vi "VI1.vi"() -> ()   [LabVIEW 2020]
uses:
  <vilib>/Utility/NIReport.llb/Report Type.ctl
  <vilib>/DAQmx/write.llb/DAQmx Write (Analog Wfm 1Chan NSamp).vi
  <vilib>/DAQmx/read.llb/DAQmx Read (Analog 1D Wfm NChan NSamp).vi
  <vilib>/DAQmx/miscellaneous.llb/DAQmx Fill In Error Info.vi
  <vilib>/measure/madcrms.llb/Basic Averaged DC-RMS for 1 Chan.vi
  <vilib>/Utility/NIReport.llb/Append Report Text (str wrap).vi
  <vilib>/measure/mascope.llb/Amplitude and Levels 1 chan.vi
  <vilib>/Utility/NIReport.llb/NI_report.lvclass
  <vilib>/measure/NI_MABase.lvlib
  <vilib>/measure/NI_MAPro.lvlib
  <vilib>/Utility/NIReport.llb/NI_ReportGenerationCore.lvlib
panel:
  in  "Tab Control 2":T1(tab)
  out "input signal":waveform(dbl)(graph)
  out "output signal":waveform(dbl)(graph)
  out "DC input":dbl format="%0.2p"
  out "RMS input":dbl format="%0.2p"
  out "DC output":dbl format="%0.2p"
  out "RMS output":dbl format="%0.2p"
  in  "amplitude 2":dbl=1.0 format="%0.2p"
  in  "rate 2":dbl=1000.0
  in  "number of samples 2":dbl=100.0
  in  "frequency":dbl=10.0 format="%0.2p"
  in  "offset":dbl format="%0.2p"
  out "iter":i32
  out "N\n 2":i32=100
  in  "(1) student ID 2":string
  in  "(1) student name  2":string
  in  "(1) student name":string
  in  "(1) student ID":string
  out "Date and time 8":string
  in  "(1) additional comment":string
  out "common gain":cluster{dbl[], dbl[]}(graph)
  out "ch 1 signal":waveform(dbl)(graph)
  out "ch 2 signal":waveform(dbl)(graph)
  in  "amplitude 3":dbl=1.0 format="%0.2p"
  in  "offset 2":dbl format="%0.2p"
  in  "Rprobe":dbl format="%0.2p"
  in  "To   [Hz]":i32
  in  "From [Hz]":dbl
  in  "jump":dbl=1.0 format="%#_13g"
  out "current freq":dbl
  in  "rate 3":dbl=1000.0
  in  "number of samples 3":dbl=100.0
  out "current jump":dbl=1.0
  out "N 4":dbl
  out "i 4":i32
  out "ch 1 input":waveform(dbl)(graph)
  out "ch 0 output":waveform(dbl)(graph)
  in  "jump [volt]":dbl=1.0 format="%#_13g"
  in  "From [volt]":dbl
  out "current amp":dbl
  in  "To   [volt]":i32
  in  "rate 7":dbl=1000.0
  in  "number of samples 7":dbl=100.0
  out "current jump 2":dbl=1.0
  in  "offset 3":dbl format="%0.2p"
  in  "frequency 2":dbl=10.0 format="%0.2p"
  out "N 7":dbl
  out "i 7":i32
  out "Vpp ch0":dbl format="%.2p"
  out "Vpp ch1":dbl format="%.2p"
  in  "stop":bool
  out "Date and time 7":string
  in  "(7) student ID 1":string
  in  "(7) student name 1":string
  in  "(7) student name 2":string
  in  "(7) student ID 2":string
  in  "(7) additional comment":string
  out "start volt 2":dbl
  # "offset measurment"
  # "function generator"
  # "Report generation"
  # "measurment details"
  # "frequency sweep"
  # "function generator"
  # "Dynamic range measurment"
  # "voltage sweep"
  # "function generator"
  # "Report generation"
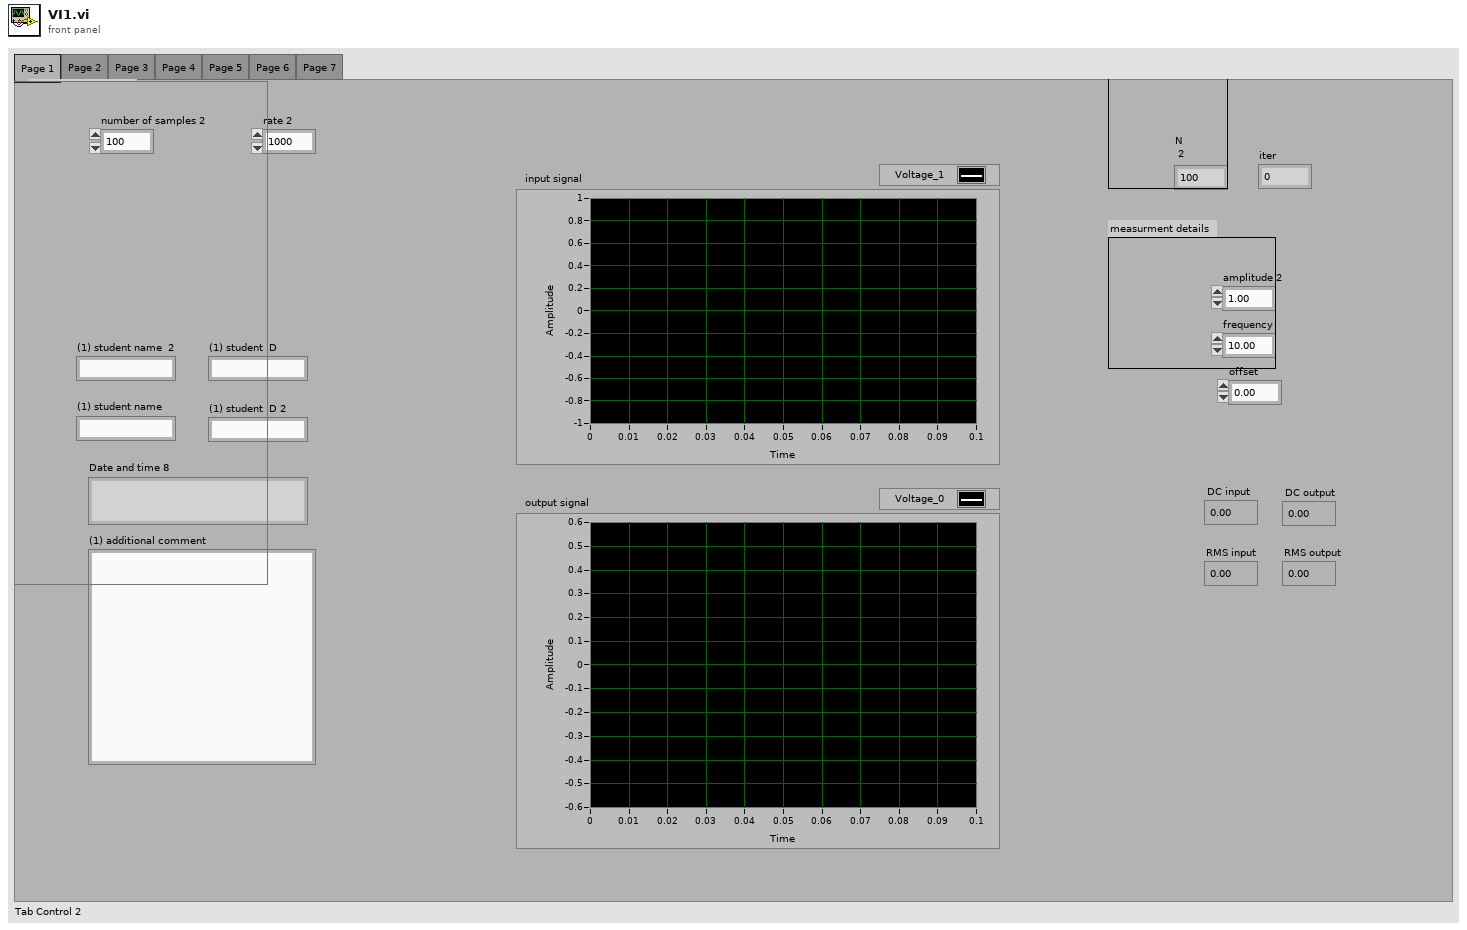
[diagram p1: front panel]
types:
  T1 = enum32{"Page 1", "Page 2", "Page 3", "Page 4", "Page 5", "Page 6", "Page 7"}
  T2 = typedef "NI_ReportGenerationCore.lvlib/Report Type.ctl" = enum16{"HTML", "Word", "Excel"}
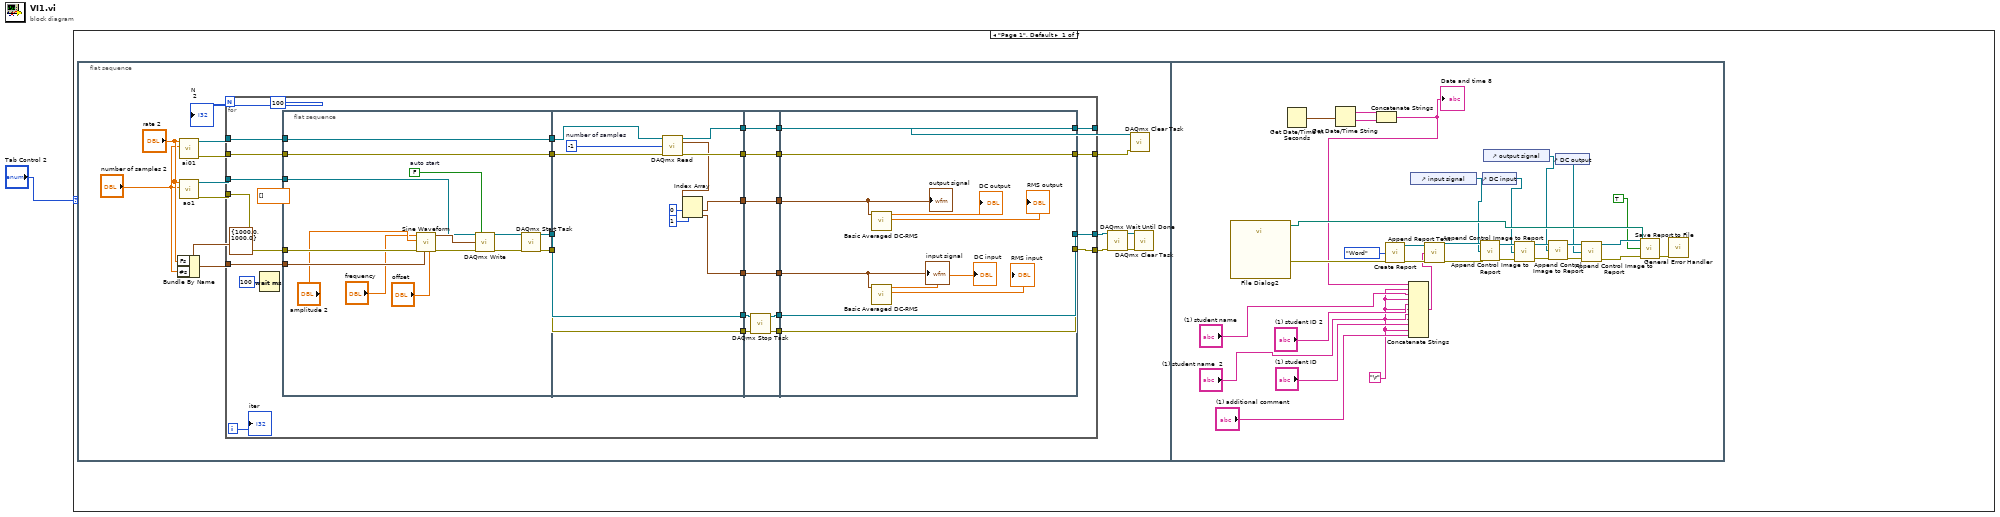
[diagram p0: block diagram]
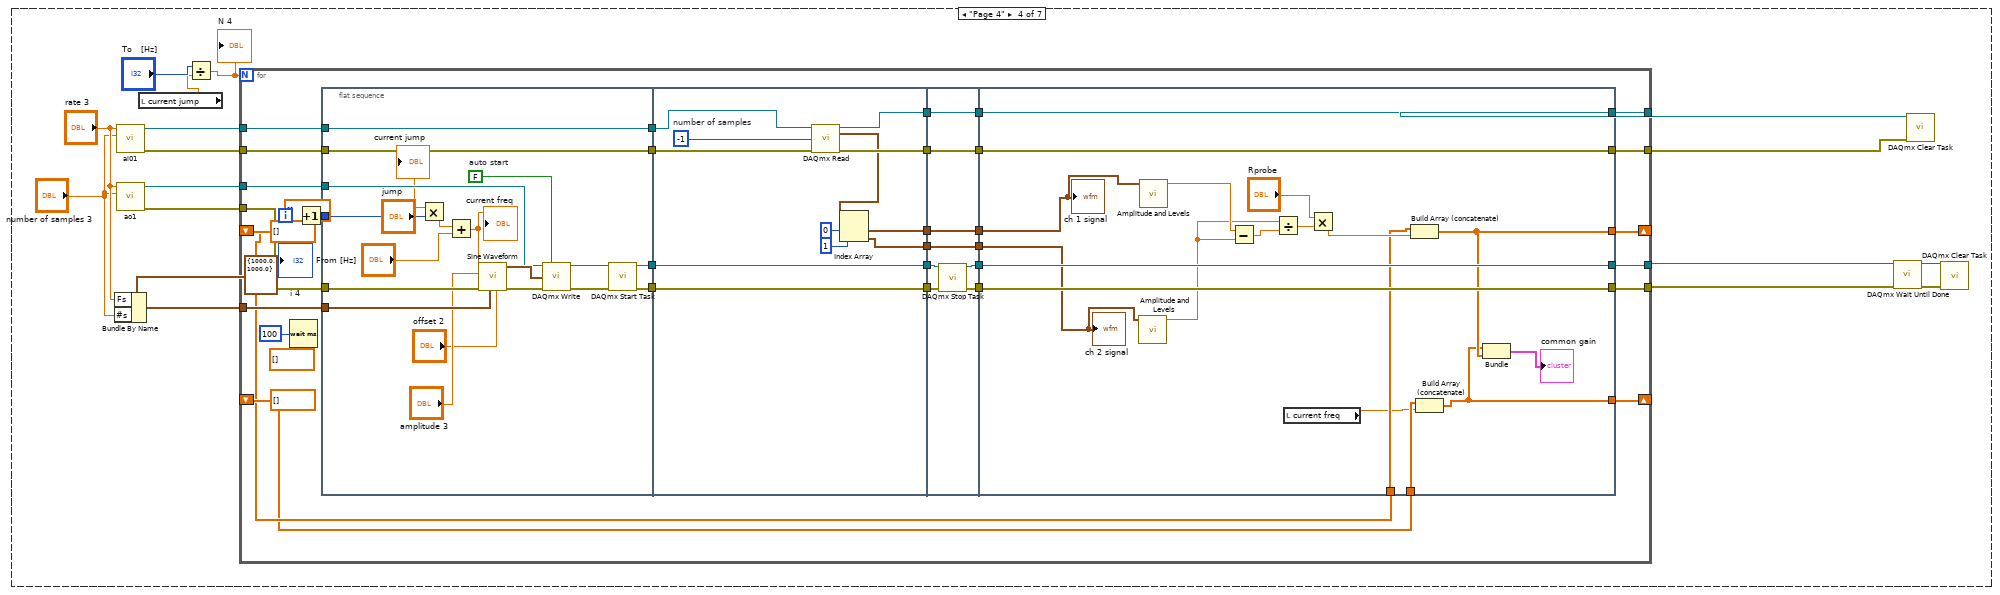
[diagram p4: hidden frame]
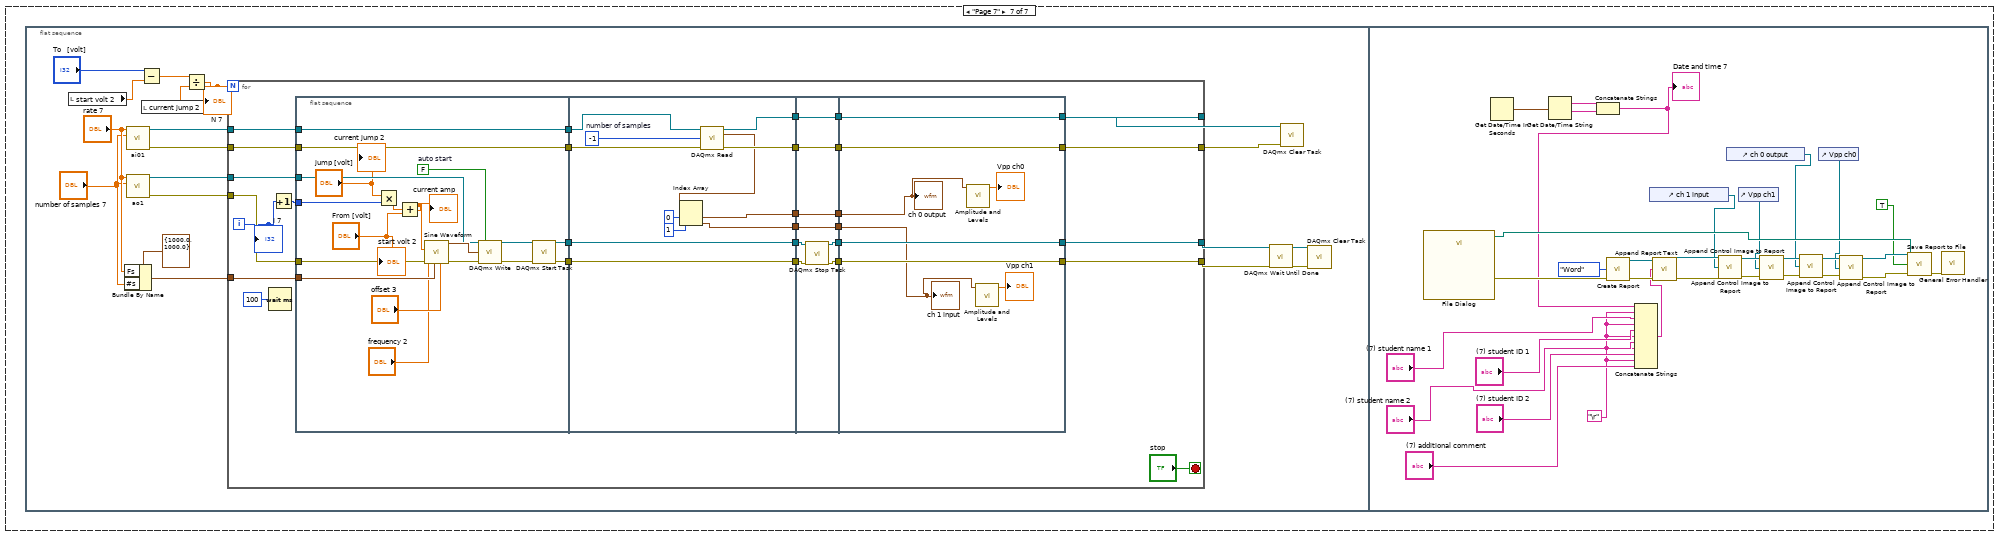
[diagram p7: hidden frame]
diagram:
  n1 = case shown="\"Page 1\", Default" "Tab Control 2" {
    frame "Page 1", Default {
      n2 = flat-sequence {
        frame #0 {
          (unwired) dbl[] []
          w10 = 100
          n3 = Bundle By Name(cluster=cluster{"Fs":dbl, "#s":dbl} {"Fs"=1000.0, "#s"=1000.0} ("sampling info"), "Fs"="rate 2", "#s"="number of samples 2") -> (w11:cluster{"Fs":dbl, "#s":dbl})
          n4 = call "ai01.vi"("number of samples"="number of samples 2", "rate"="rate 2") -> ("error out"=w6:errorcluster, "task out"=w7:refnum<k21>)  [unwired: 8 in]
          n5 = call "ao1.vi"("number of samples"="number of samples 2", "rate"="rate 2") -> ("error out"=w14:errorcluster, "task out"=w13:refnum<k21>)  [unwired: 8 in]
          n6 = for {
            N: w10 -> [_]
            tunnel: w14 -> [w43]
            tunnel: w13 -> [w42]
            tunnel: w11 -> [w41]
            tunnel: [w40] -> w9
            tunnel: [w39] -> w8
            tunnel: w7 -> [w38]
            tunnel: w6 -> [w36]
            tunnel: [w33] -> w3
            tunnel: [w31] -> w2
            i -> [w17]
            n7 = Wait (ms)(milliseconds to wait=u32 100) -> ()  [unwired: 1 out]
            n8 = flat-sequence {
              tunnel: w43 -> [w55]
              tunnel: w42 -> [w54]
              tunnel: w41 -> [w53]
              tunnel: w38 -> [w49]
              tunnel: [w49] -> w37
              tunnel: w36 -> [w48]
              tunnel: [w48] -> w35
              tunnel: [w47] -> w29
              tunnel: [w46] -> w27
              tunnel: w37 -> [w69]
              tunnel: w35 -> [w68]
              tunnel: [w67] -> w34
              tunnel: [w66] -> w32
              tunnel: [w65] -> w30
              tunnel: w29 -> [w65]
              tunnel: [w64] -> w28
              tunnel: w27 -> [w64]
              tunnel: [w60] -> w20
              tunnel: [w59] -> w18
              tunnel: w34 -> [w76]
              tunnel: w32 -> [w75]
              tunnel: w30 -> [w74]
              tunnel: w28 -> [w73]
              tunnel: [w78] -> w25
              tunnel: [w77] -> w24
              tunnel: [w76] -> w23
              tunnel: [w75] -> w22
              tunnel: [w72] -> w21
              tunnel: w20 -> [w72]
              tunnel: [w71] -> w19
              tunnel: w18 -> [w71]
              tunnel: [w85] -> w31
              tunnel: [w86] -> w33
              tunnel: [w87] -> w39
              tunnel: [w88] -> w40
              tunnel: w25 -> [w88]
              tunnel: w24 -> [w87]
              tunnel: w23 -> [w86]
              tunnel: w22 -> [w85]
              tunnel: w21 -> [w84]
              tunnel: w19 -> [w83]
              frame #0 {
                w58 = FALSE  # auto start
                n9 = call <vilib>:"Sine Waveform.vi"("offset"="offset", "sampling info"=w53, "error in (no error)"=w55, "amplitude"="amplitude 2", "frequency"="frequency") -> ("error out"=w57:errorcluster, "signal out"=w56:waveform(dbl))  [unwired: 5 in]
                n10 = call-poly <vilib>:"DAQmx Write.vi"("task/channels in"=w54, "auto start"=w58, "data"=w56, "error in"=w57) -> ("task out"=w51:refnum<k21>, "error out"=w50:errorcluster)  [unwired: 9 in, 1 out]
                n11 = call <vilib>:"DAQmx Start Task.vi"("task/channels in"=w51, "error in"=w50) -> ("task out"=w47:refnum<k21>, "error out"=w46:errorcluster)  [unwired: 12 in]
              }
              frame #1 {
                w70 = -1  # number of samples
                n12 = call-poly <vilib>:"DAQmx Read.vi"("task/channels in"=w69, "number of samples per channel"=w70, "error in"=w68) -> ("task out"=w67:refnum<k21>, "data"=w63:waveform(dbl)[], "error out"=w66:errorcluster)  [unwired: 10 in]
                n13 = Index Array(array=w63, index #1=0 ("index"), index #2=1 ("index")) -> (element #1=w60:waveform(dbl), element #2=w59:waveform(dbl))
              }
              frame #2 {
                n14 = call <vilib>:"DAQmx Stop Task.vi"("task/channels in"=w74, "error in"=w73) -> ("task out"=w78:refnum<k21>, "error out"=w77:errorcluster)  [unwired: 12 in]
              }
              frame #3 {
                n15 = call-poly <vilib>:"Basic Averaged DC-RMS.vi"("signal in"=w84) -> ("RMS value"=→"RMS output":dbl, "DC value"=→"DC output":dbl)  [unwired: 7 in, 2 out]
                n16 = call-poly <vilib>:"Basic Averaged DC-RMS.vi"("signal in"=w83) -> ("RMS value"=→"RMS input":dbl, "DC value"=→"DC input":dbl)  [unwired: 7 in, 2 out]
                "output signal" <- w84
                "input signal" <- w83
              }
            }
            "iter" <- w17
          }
          n17 = call <vilib>:"DAQmx Wait Until Done.vi"("task/channels in"=w9, "error in"=w8) -> ("task out"=w15:refnum<k21>, "error out"=w16:errorcluster)  [unwired: 12 in]
          n18 = call <vilib>:"DAQmx Clear Task.vi"("task in"=w3, "error in"=w2) -> ()  [unwired: 13 in, 1 out]
          n19 = call <vilib>:"DAQmx Clear Task.vi"("task in"=w15, "error in"=w16) -> ()  [unwired: 13 in, 1 out]
          "N\n 2" <- w10
        }
        frame #1 {
          w105 = "\r"
          n20 = call "File Dialog2"() -> ("selected path"=w108:path, "error out"=w107:errorcluster)  [unwired: 12 in, 2 out]
          n21 = Get Date/Time In Seconds() -> (seconds since 1Jan1904=w120:timestamp)
          n22 = Get Date/Time String(seconds (now)=w120) -> (date string=w118:string, time string=w119:string)  [unwired: 2 in]
          n23 = Concatenate Strings(w118, w119) -> (w103:string)
          "Date and time 8" <- w103
          n24 = call <vilib>:"Create Report.vi"("report type"=Report_Type."Word", "error in (no error)"=w107) -> ("report out"=w109:refnum<class "NI_report.lvclass">, "error out"=w111:errorcluster)  [unwired: 12 in]
          n25 = Concatenate Strings(w103, w105, "(1) student name", w105, "(1) student ID 2", w105, "(1) student name  2", w105, "(1) student ID", w105, "(1) additional comment") -> (w101:string)
          n26 = control-ref of="input signal"() -> (w92:refnum<vi>)
          n27 = call-poly <vilib>:"Append Report Text.vi"("report in"=w109, "text"=w101, "error in (no error)"=w111) -> ("report out"=w94:refnum<class "NI_report.lvclass">, "error out"=w93:errorcluster)  [unwired: 9 in, 2 out]
          n28 = call-dynamic "Append Control Image to Report.vi"("report in"=w94, "ctrl reference"=w92, "error in (no error)"=w93) -> ("report out"=w96:refnum<class "NI_report.lvclass">, "error out"=w95:errorcluster)  [unwired: 9 in, 2 out]
          n29 = control-ref of="DC input"() -> (w91:refnum<vi>)
          n30 = control-ref of="output signal"() -> (w90:refnum<vi>)
          n31 = call-dynamic "Append Control Image to Report.vi"("report in"=w96, "ctrl reference"=w91, "error in (no error)"=w95) -> ("report out"=w97:refnum<class "NI_report.lvclass">, "error out"=w98:errorcluster)  [unwired: 9 in, 2 out]
          n32 = call-dynamic "Append Control Image to Report.vi"("report in"=w97, "ctrl reference"=w90, "error in (no error)"=w98) -> ("report out"=w100:refnum<class "NI_report.lvclass">, "error out"=w99:errorcluster)  [unwired: 9 in, 2 out]
          n33 = control-ref of="DC output"() -> (w89:refnum<vi>)
          n34 = call-dynamic "Append Control Image to Report.vi"("report in"=w100, "ctrl reference"=w89, "error in (no error)"=w99) -> ("report out"=w110:refnum<class "NI_report.lvclass">, "error out"=w112:errorcluster)  [unwired: 9 in, 2 out]
          n35 = call-dynamic "Save Report to File.vi"("report in"=w110, "report file path"=w108, "prompt to replace? (F)"=TRUE, "error in (no error)"=w112) -> ("error out"=w102:errorcluster)  [unwired: 10 in, 1 out]
          n36 = call <vilib>:"General Error Handler.vi"("error in (no error)"=w102) -> ()  [unwired: 10 in, 5 out]
        }
      }
    }
    frame "Page 2" {
    }
    frame "Page 3" {
    }
    frame "Page 4" {
      (unwired) dbl[] []
      (unwired) dbl[] []
      n37 = Bundle By Name(cluster=cluster{"Fs":dbl, "#s":dbl} {"Fs"=1000.0, "#s"=1000.0} ("sampling info"), "Fs"="rate 3", "#s"="number of samples 3") -> (w136:cluster{"Fs":dbl, "#s":dbl})
      n38 = call "ai01.vi"("number of samples"="number of samples 3", "rate"="rate 3") -> ("error out"=w134:errorcluster, "task out"=w135:refnum<k21>)  [unwired: 8 in]
      n39 = call "ao1.vi"("number of samples"="number of samples 3", "rate"="rate 3") -> ("error out"=w139:errorcluster, "task out"=w138:refnum<k21>)  [unwired: 8 in]
      n40 = local read "current jump"() -> (w125:dbl)
      n41 = Divide(x="To   [Hz]", y=w125) -> (x/y=w127:dbl)
      "N 4" <- w127
      n42 = for {
        N: w127 -> [_]
        tunnel: w139 -> [w171]
        tunnel: w138 -> [w170]
        tunnel: w136 -> [w167]
        tunnel: [w166] -> w122
        tunnel: [w165] -> w121
        tunnel: w135 -> [w164]
        tunnel: w134 -> [w162]
        tunnel: [w159] -> w131
        tunnel: [w157] -> w130
        shift-right: [w143] -> _
        shift-left: dbl[] [] -> [w142]
        shift-right: [w141] -> _
        shift-left: dbl[] [] -> [w140]
        i -> [w169]
        n43 = Wait (ms)(milliseconds to wait=u32 100) -> ()  [unwired: 1 out]
        n44 = Increment(x=w169) -> (x+1=w168:i32)
        n45 = flat-sequence {
          tunnel: w171 -> [w187]
          tunnel: w170 -> [w186]
          tunnel: w168 -> [w175]
          tunnel: w167 -> [w184]
          tunnel: w164 -> [w181]
          tunnel: [w181] -> w163
          tunnel: w162 -> [w180]
          tunnel: [w180] -> w161
          tunnel: [w179] -> w155
          tunnel: [w178] -> w153
          tunnel: w163 -> [w201]
          tunnel: w161 -> [w200]
          tunnel: [w199] -> w160
          tunnel: [w198] -> w158
          tunnel: [w197] -> w156
          tunnel: w155 -> [w197]
          tunnel: [w196] -> w154
          tunnel: w153 -> [w196]
          tunnel: [w192] -> w146
          tunnel: [w191] -> w145
          tunnel: w160 -> [w208]
          tunnel: w158 -> [w207]
          tunnel: w156 -> [w206]
          tunnel: w154 -> [w205]
          tunnel: [w210] -> w151
          tunnel: [w209] -> w150
          tunnel: [w208] -> w149
          tunnel: [w207] -> w148
          tunnel: [w204] -> w147
          tunnel: w146 -> [w204]
          tunnel: w145 -> [w203]
          tunnel: [w203] -> w144
          tunnel: [w225] -> w157
          tunnel: [w226] -> w159
          tunnel: [w227] -> w165
          tunnel: [w228] -> w166
          tunnel: w151 -> [w228]
          tunnel: w150 -> [w227]
          tunnel: w149 -> [w226]
          tunnel: w148 -> [w225]
          tunnel: w147 -> [w223]
          tunnel: w144 -> [w224]
          tunnel: [w217] -> w143
          tunnel: w142 -> [w218]
          tunnel: [w214] -> w141
          tunnel: w140 -> [w216]
          frame #0 {
            w190 = FALSE  # auto start
            n46 = Multiply(x="jump", y=w175) -> (x*y=w174:dbl)
            n47 = Add(x=w174, y="From [Hz]") -> (x+y=w173:dbl)
            "current freq" <- w173
            n48 = call <vilib>:"Sine Waveform.vi"("offset"="offset 2", "sampling info"=w184, "error in (no error)"=w187, "amplitude"="amplitude 3", "frequency"=w173) -> ("error out"=w189:errorcluster, "signal out"=w188:waveform(dbl))  [unwired: 5 in]
            n49 = call-poly <vilib>:"DAQmx Write.vi"("task/channels in"=w186, "auto start"=w190, "data"=w188, "error in"=w189) -> ("task out"=w183:refnum<k21>, "error out"=w182:errorcluster)  [unwired: 9 in, 1 out]
            n50 = call <vilib>:"DAQmx Start Task.vi"("task/channels in"=w183, "error in"=w182) -> ("task out"=w179:refnum<k21>, "error out"=w178:errorcluster)  [unwired: 12 in]
            "current jump" <- "jump"
          }
          frame #1 {
            w202 = -1  # number of samples
            n51 = call-poly <vilib>:"DAQmx Read.vi"("task/channels in"=w201, "number of samples per channel"=w202, "error in"=w200) -> ("task out"=w199:refnum<k21>, "data"=w195:waveform(dbl)[], "error out"=w198:errorcluster)  [unwired: 10 in]
            n52 = Index Array(array=w195, index #1=0 ("index"), index #2=1 ("index")) -> (element #1=w192:waveform(dbl), element #2=w191:waveform(dbl))
          }
          frame #2 {
            n53 = call <vilib>:"DAQmx Stop Task.vi"("task/channels in"=w206, "error in"=w205) -> ("task out"=w210:refnum<k21>, "error out"=w209:errorcluster)  [unwired: 12 in]
          }
          frame #3 {
            n54 = call-poly <vilib>:"Amplitude and Levels.vi"("signal in"=w224) -> ("amplitude"=w211:dbl)  [unwired: 7 in, 3 out]
            n55 = call-poly <vilib>:"Amplitude and Levels.vi"("signal in"=w223) -> ("amplitude"=w212:dbl)  [unwired: 7 in, 3 out]
            n56 = Subtract(x=w212, y=w211) -> (x-y=w222:dbl)
            n57 = Divide(x=w211, y=w222) -> (x/y=w221:dbl)
            n58 = local read "current freq"() -> (w215:dbl)
            n59 = Multiply(x="Rprobe", y=w221) -> (x*y=w219:dbl)
            n60 = Build Array (concatenate)(w218, w219) -> (w217:dbl[])
            n61 = Build Array (concatenate)(w216, w215) -> (w214:dbl[])
            n62 = Bundle(w214, w217) -> (→"common gain":cluster{dbl[], dbl[]})  [unwired: 1 in]
            "ch 1 signal" <- w223
            "ch 2 signal" <- w224
          }
        }
        "i 4" <- w169
      }
      n63 = call <vilib>:"DAQmx Wait Until Done.vi"("task/channels in"=w122, "error in"=w121) -> ("task out"=w124:refnum<k21>, "error out"=w123:errorcluster)  [unwired: 12 in]
      n64 = call <vilib>:"DAQmx Clear Task.vi"("task in"=w131, "error in"=w130) -> ()  [unwired: 13 in, 1 out]
      n65 = call <vilib>:"DAQmx Clear Task.vi"("task in"=w124, "error in"=w123) -> ()  [unwired: 13 in, 1 out]
    }
    frame "Page 5" {
    }
    frame "Page 6" {
    }
    frame "Page 7" {
      n66 = flat-sequence {
        frame #0 {
          n67 = local read "start volt 2"() -> (w229:dbl)
          n68 = Bundle By Name(cluster=cluster{"Fs":dbl, "#s":dbl} {"Fs"=1000.0, "#s"=1000.0} ("sampling info"), "Fs"="rate 7", "#s"="number of samples 7") -> (w244:cluster{"Fs":dbl, "#s":dbl})
          n69 = call "ai01.vi"("number of samples"="number of samples 7", "rate"="rate 7") -> ("error out"=w242:errorcluster, "task out"=w243:refnum<k21>)  [unwired: 8 in]
          n70 = call "ao1.vi"("number of samples"="number of samples 7", "rate"="rate 7") -> ("error out"=w247:errorcluster, "task out"=w246:refnum<k21>)  [unwired: 8 in]
          n71 = Subtract(x="To   [volt]", y=w229) -> (x-y=w231:dbl)
          n72 = local read "current jump 2"() -> (w230:dbl)
          n73 = Divide(x=w231, y=w230) -> (x/y=w237:dbl)
          "N 7" <- w237
          n74 = for {
            N: w237 -> [_]
            tunnel: w247 -> [w276]
            tunnel: w246 -> [w275]
            tunnel: w244 -> [w272]
            tunnel: [w271] -> w234
            tunnel: [w270] -> w233
            tunnel: w243 -> [w269]
            tunnel: w242 -> [w267]
            tunnel: [w264] -> w239
            tunnel: [w262] -> w238
            i -> [w274]
            stop <- "stop" stop-if-true
            n75 = Wait (ms)(milliseconds to wait=u32 100) -> ()  [unwired: 1 out]
            n76 = Increment(x=w274) -> (x+1=w273:i32)
            n77 = flat-sequence {
              tunnel: w276 -> [w292]
              tunnel: w275 -> [w291]
              tunnel: w273 -> [w281]
              tunnel: w272 -> [w289]
              tunnel: w269 -> [w286]
              tunnel: [w286] -> w268
              tunnel: w267 -> [w285]
              tunnel: [w285] -> w266
              tunnel: [w284] -> w260
              tunnel: [w283] -> w258
              tunnel: w268 -> [w306]
              tunnel: w266 -> [w305]
              tunnel: [w304] -> w265
              tunnel: [w303] -> w263
              tunnel: [w302] -> w261
              tunnel: w260 -> [w302]
              tunnel: [w301] -> w259
              tunnel: w258 -> [w301]
              tunnel: [w297] -> w251
              tunnel: [w296] -> w250
              tunnel: w265 -> [w313]
              tunnel: w263 -> [w312]
              tunnel: w261 -> [w311]
              tunnel: w259 -> [w310]
              tunnel: [w315] -> w256
              tunnel: [w314] -> w255
              tunnel: [w313] -> w254
              tunnel: [w312] -> w253
              tunnel: [w309] -> w252
              tunnel: w251 -> [w309]
              tunnel: w250 -> [w308]
              tunnel: [w308] -> w249
              tunnel: [w320] -> w262
              tunnel: [w321] -> w264
              tunnel: [w322] -> w270
              tunnel: [w323] -> w271
              tunnel: w256 -> [w323]
              tunnel: w255 -> [w322]
              tunnel: w254 -> [w321]
              tunnel: w253 -> [w320]
              tunnel: w252 -> [w318]
              tunnel: w249 -> [w319]
              frame #0 {
                w295 = FALSE  # auto start
                n78 = Multiply(x="jump [volt]", y=w281) -> (x*y=w280:dbl)
                n79 = Add(x=w280, y="From [volt]") -> (x+y=w278:dbl)
                "current amp" <- w278
                n80 = call <vilib>:"Sine Waveform.vi"("offset"="offset 3", "sampling info"=w289, "error in (no error)"=w292, "amplitude"=w278, "frequency"="frequency 2") -> ("error out"=w294:errorcluster, "signal out"=w293:waveform(dbl))  [unwired: 5 in]
                n81 = call-poly <vilib>:"DAQmx Write.vi"("task/channels in"=w291, "auto start"=w295, "data"=w293, "error in"=w294) -> ("task out"=w288:refnum<k21>, "error out"=w287:errorcluster)  [unwired: 9 in, 1 out]
                n82 = call <vilib>:"DAQmx Start Task.vi"("task/channels in"=w288, "error in"=w287) -> ("task out"=w284:refnum<k21>, "error out"=w283:errorcluster)  [unwired: 12 in]
                "current jump 2" <- "jump [volt]"
                "start volt 2" <- "From [volt]"
              }
              frame #1 {
                w307 = -1  # number of samples
                n83 = call-poly <vilib>:"DAQmx Read.vi"("task/channels in"=w306, "number of samples per channel"=w307, "error in"=w305) -> ("task out"=w304:refnum<k21>, "data"=w300:waveform(dbl)[], "error out"=w303:errorcluster)  [unwired: 10 in]
                n84 = Index Array(array=w300, index #1=0 ("index"), index #2=1 ("index")) -> (element #1=w297:waveform(dbl), element #2=w296:waveform(dbl))
              }
              frame #2 {
                n85 = call <vilib>:"DAQmx Stop Task.vi"("task/channels in"=w311, "error in"=w310) -> ("task out"=w315:refnum<k21>, "error out"=w314:errorcluster)  [unwired: 12 in]
              }
              frame #3 {
                n86 = call-poly <vilib>:"Amplitude and Levels.vi"("signal in"=w318) -> ("amplitude"=→"Vpp ch0":dbl)  [unwired: 7 in, 3 out]
                n87 = call-poly <vilib>:"Amplitude and Levels.vi"("signal in"=w319) -> ("amplitude"=→"Vpp ch1":dbl)  [unwired: 7 in, 3 out]
                "ch 0 output" <- w318
                "ch 1 input" <- w319
              }
            }
            "i 7" <- w274
          }
          n88 = call <vilib>:"DAQmx Wait Until Done.vi"("task/channels in"=w234, "error in"=w233) -> ("task out"=w236:refnum<k21>, "error out"=w235:errorcluster)  [unwired: 12 in]
          n89 = call <vilib>:"DAQmx Clear Task.vi"("task in"=w239, "error in"=w238) -> ()  [unwired: 13 in, 1 out]
          n90 = call <vilib>:"DAQmx Clear Task.vi"("task in"=w236, "error in"=w235) -> ()  [unwired: 13 in, 1 out]
        }
        frame #1 {
          w340 = "\r"
          n91 = call "File Dialog"() -> ("selected path"=w343:path, "error out"=w342:errorcluster)  [unwired: 12 in, 2 out]
          n92 = Get Date/Time In Seconds() -> (seconds since 1Jan1904=w355:timestamp)
          n93 = Get Date/Time String(seconds (now)=w355) -> (date string=w353:string, time string=w354:string)  [unwired: 2 in]
          n94 = Concatenate Strings(w353, w354) -> (w338:string)
          "Date and time 7" <- w338
          n95 = call <vilib>:"Create Report.vi"("report type"=Report_Type."Word", "error in (no error)"=w342) -> ("report out"=w344:refnum<class "NI_report.lvclass">, "error out"=w346:errorcluster)  [unwired: 12 in]
          n96 = Concatenate Strings(w338, w340, "(7) student name 1", w340, "(7) student ID 1", w340, "(7) student name 2", w340, "(7) student ID 2", w340, "(7) additional comment") -> (w336:string)
          n97 = control-ref of="ch 1 input"() -> (w327:refnum<vi>)
          n98 = call-poly <vilib>:"Append Report Text.vi"("report in"=w344, "text"=w336, "error in (no error)"=w346) -> ("report out"=w329:refnum<class "NI_report.lvclass">, "error out"=w328:errorcluster)  [unwired: 9 in, 2 out]
          n99 = call-dynamic "Append Control Image to Report.vi"("report in"=w329, "ctrl reference"=w327, "error in (no error)"=w328) -> ("report out"=w331:refnum<class "NI_report.lvclass">, "error out"=w330:errorcluster)  [unwired: 9 in, 2 out]
          n100 = control-ref of="ch 0 output"() -> (w325:refnum<vi>)
          n101 = control-ref of="Vpp ch1"() -> (w326:refnum<vi>)
          n102 = call-dynamic "Append Control Image to Report.vi"("report in"=w331, "ctrl reference"=w326, "error in (no error)"=w330) -> ("report out"=w332:refnum<class "NI_report.lvclass">, "error out"=w333:errorcluster)  [unwired: 9 in, 2 out]
          n103 = call-dynamic "Append Control Image to Report.vi"("report in"=w332, "ctrl reference"=w325, "error in (no error)"=w333) -> ("report out"=w335:refnum<class "NI_report.lvclass">, "error out"=w334:errorcluster)  [unwired: 9 in, 2 out]
          n104 = control-ref of="Vpp ch0"() -> (w324:refnum<vi>)
          n105 = call-dynamic "Append Control Image to Report.vi"("report in"=w335, "ctrl reference"=w324, "error in (no error)"=w334) -> ("report out"=w345:refnum<class "NI_report.lvclass">, "error out"=w347:errorcluster)  [unwired: 9 in, 2 out]
          n106 = call-dynamic "Save Report to File.vi"("report in"=w345, "report file path"=w343, "prompt to replace? (F)"=TRUE, "error in (no error)"=w347) -> ("error out"=w337:errorcluster)  [unwired: 10 in, 1 out]
          n107 = call <vilib>:"General Error Handler.vi"("error in (no error)"=w337) -> ()  [unwired: 10 in, 5 out]
        }
      }
    }
  }
